vi "PCOM串口调试助手.vi"() -> ()   [LabVIEW 2019]
panel:
  in  "选项卡控件":enum32{"串口设置", "图形显示"}(tab)
  in  "串口设置":T1={"波特率"=9600, "数据位"=8, "校验"=enum."None", "停止位"=10, "VISA资源名称"="COM1", "XON"=enum."DC1", "XOFF"=enum."DC3", "终止符时结束读取？"=TRUE, "终止符"=10, "流控制"=0} {"流控制" items=["无"=0, "XON/XOFF"=1, "RTS/CTS"=2, "DTR/DSR"=4]; "终止符" format="%.0x"; "停止位" items=["1.0"=10, "1.5"=15, "2.0"=20]; "数据位" min=5 max=8 step=1; "波特率" items=["75"=75, "110"=110, "134"=134, "150"=150, "300"=300, "600"=600, "1200"=1200, "1800"=1800, "2400"=2400, "4800"=4800, "7200"=7200, "9600"=9600, "14400"=14400, "19200"=19200, "28800"=28800, "38400"=38400, "56000"=56000, "57600"=57600, "115200"=115200, "128000"=128000, "230400"=230400]}
  out "接受字符串":string
  in  "停止":bool
  in  "打开串口":bool
  in  "写入簇":cluster{"命令":string, "是否写入":bool}={"命令"="*IDN?", "是否写入"=FALSE}
  out "波形图表":dbl(graph)
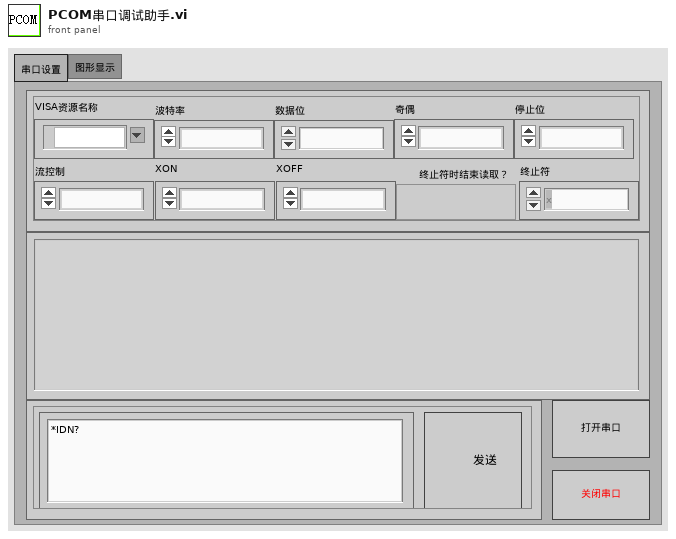
[diagram p1: front panel]
types:
  T1 = cluster{"波特率":u32, "数据位":u16, "校验":enum16{"None", "Odd", "Even", "Mark", "Space"}, "停止位":u16, "VISA资源名称":refnum<visa-resource-name>, "XON":enum16{"NUL", "SOH", "STX", "ETX", "EOT", "ENQ", "ACK", "BEL", "BS", "HT", "LF", "VT", "FF", "CR", "SO", "SI", "DLE", "DC1", "DC2", "DC3", "DC4", "NAK", "SYN", "ETB", "CAN", "EM", "SUB", "ESC", "FS", "GS", "RS", "US", "SP", "!", "\"", "#", "$", "%", "&", "'", "(", ")", "*", "+", ",", "- (-)", ".", "/", "0", "1", "2", "3", "4", "5", "6", "7", "8", "9", ":", ";", "<", "=", ">", "?", "@", "A", "B", "C", "D", "E", "F", "G", "H", "I", "J", "K", "L", "M", "N", "O", "P", "Q", "R", "S", "T", "U", "V", "W", "X", "Y", "Z", "[", "\\", "]", "^", "_", "`", "a", "b", "c", "d", "e", "f", "g", "h", "i", "j", "k", "l", "m", "n", "o", "p", "q", "r", "s", "t", "u", "v", "w", "x", "y", "z", "{", "|", "}", "~"}, "XOFF":enum16{"NUL", "SOH", "STX", "ETX", "EOT", "ENQ", "ACK", "BEL", "BS", "HT", "LF", "VT", "FF", "CR", "SO", "SI", "DLE", "DC1", "DC2", "DC3", "DC4", "NAK", "SYN", "ETB", "CAN", "EM", "SUB", "ESC", "FS", "GS", "RS", "US", "SP", "!", "\"", "#", "$", "%", "&", "'", "(", ")", "*", "+", ",", "- (-)", ".", "/", "0", "1", "2", "3", "4", "5", "6", "7", "8", "9", ":", ";", "<", "=", ">", "?", "@", "A", "B", "C", "D", "E", "F", "G", "H", "I", "J", "K", "L", "M", "N", "O", "P", "Q", "R", "S", "T", "U", "V", "W", "X", "Y", "Z", "[", "\\", "]", "^", "_", "`", "a", "b", "c", "d", "e", "f", "g", "h", "i", "j", "k", "l", "m", "n", "o", "p", "q", "r", "s", "t", "u", "v", "w", "x", "y", "z", "{", "|", "}", "~"}, "终止符时结束读取？":bool, "终止符":u8, "流控制":u16}
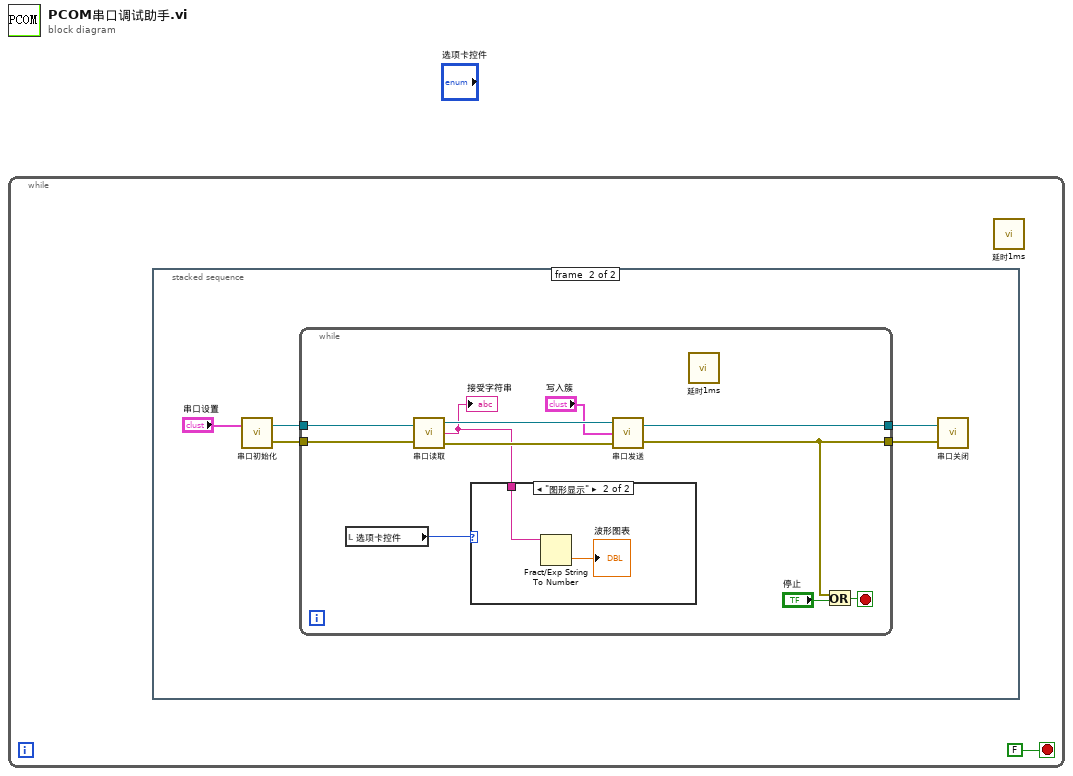
[diagram p0: block diagram]
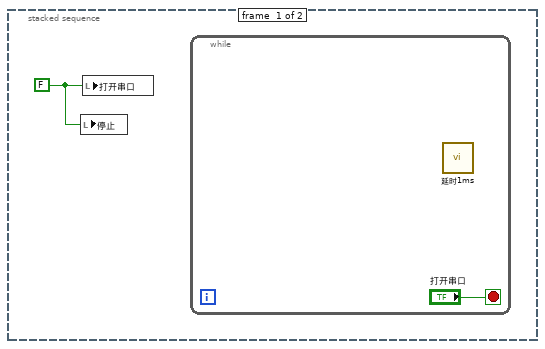
[diagram p2: hidden frame]
diagram:
  n1 = while {
    stop <- FALSE stop-if-true
    n2 = stacked-sequence {
      frame #0 {
        w2 = FALSE ("打开串口")
        n3 = local write "停止"(w2) -> ()
        n4 = local write "打开串口"(w2) -> ()
        n5 = while {
          stop <- "打开串口" stop-if-true
          n6 = call "延时1ms.vi"() -> ()  [unwired: 12 in]
        }
      }
      frame #1 {
        n7 = call "串口初始化.vi"("串口设置"="串口设置") -> ("错误输出"=w6:errorcluster, "VISA resource name out"=w5:refnum<visa-resource-name>)  [unwired: 1 in]
        n8 = while {
          tunnel: [w19] -> w7
          tunnel: w6 -> [w18]
          tunnel: w5 -> [w17]
          tunnel: [w15] -> w4
          stop <- w14 stop-if-true
          n9 = local read "选项卡控件"() -> (w9:enum32{"串口设置", "图形显示"})
          n10 = call "串口读取.vi"("VISA resource name in"=w17, "错误输入（无错误）"=w18) -> ("VISA resource name out"=w12:refnum<visa-resource-name>, "响应"=w10:string, "错误输出"=w13:errorcluster)
          "接受字符串" <- w10
          n11 = case shown="\"图形显示\"" w9 {
            tunnel: w10 -> [_ w21]
            frame "串口设置", Default {
            }
            frame "图形显示" {
              n12 = Fract/Exp String To Number(string=w21) -> (number=→"波形图表":dbl)  [unwired: 3 in, 1 out]
            }
          }
          n13 = call "串口发送.vi"("错误输入（无错误）"=w13, "写入配置"="写入簇", "VISA resource name in"=w12) -> ("错误输出"=w15:errorcluster, "VISA resource name out"=w19:refnum<visa-resource-name>)
          n14 = call "延时1ms.vi"() -> ()  [unwired: 12 in]
          n15 = Or(x=w15, y="停止") -> (x .or. y?=w14:bool)
        }
        n16 = call "串口关闭.vi"("错误输入（无错误）"=w4, "VISA资源名称"=w7) -> ()  [unwired: 1 in]
      }
    }
    n17 = call "延时1ms.vi"() -> ()  [unwired: 12 in]
  }
